vi "ProgramGS200andRun.vi"(5 "error in":errorcluster, 6 "Run program?":bool, 7 "Interval input":dbl, 8 "Slope Input":dbl, 9 "Voltage array":dbl[](array[numeric]), 10 "VISA resource name":refnum<visa-resource-name>) -> (0 "error out":errorcluster, 3 "VISA resource name out":refnum<visa-resource-name>)   [LabVIEW 2019]
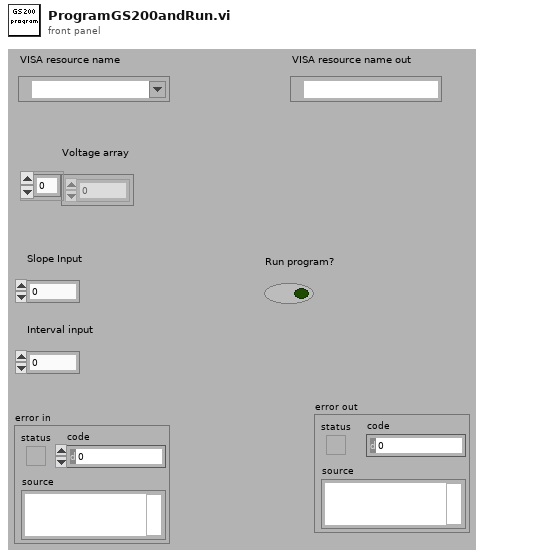
[diagram p1: front panel]
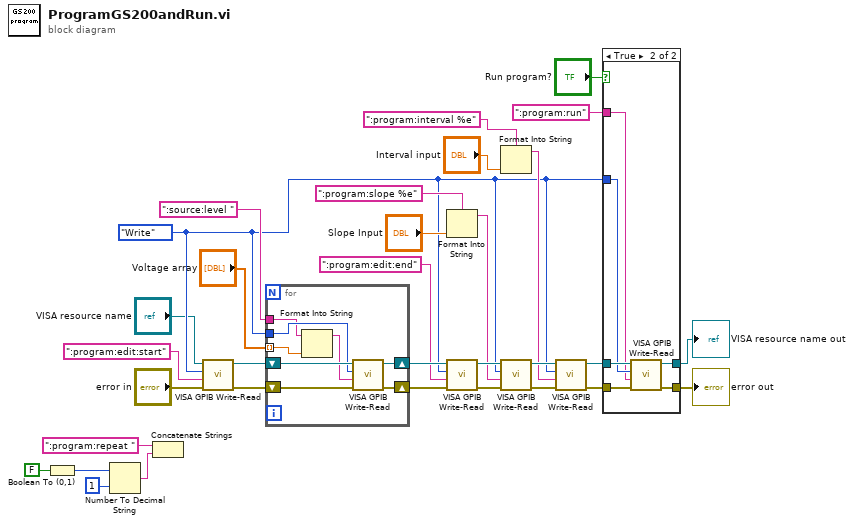
[diagram p0: block diagram]
diagram:
  w5 = enum16{"Write", "Read", "Write & Read"}."Write" ("Action")
  n1 = Boolean To (0,1)(Boolean=FALSE ("Repeat program?")) -> (0, 1=w25:i16)
  n2 = Number To Decimal String(number=w25, width (-)=i16 1) -> (decimal integer string=w22:string)
  n3 = Concatenate Strings(":program:repeat ", w22) -> ()  [unwired: 1 out]
  n4 = call "VISA GPIB Write-Read.vi"("error in (no error)"="error in", "Command"=":program:edit:start", "Action"=w5, "VISA resource name"="VISA resource name") -> ("error out"=w19:errorcluster, "dup VISA Session"=w20:refnum<visa-resource-name>)  [unwired: 4 in, 2 out]
  n5 = for {
    tunnel: ":source:level " -> [w36]
    tunnel: w5 -> [w38]
    tunnel: "Voltage array" -> [w35] mode=indexing
    shift-right: [w34] -> w15
    shift-left: w19 -> [w39]
    shift-right: [w33] -> w16
    shift-left: w20 -> [w40]
    n6 = Format Into String(initial string=w36, w35) -> (resulting string=w37:string)  [unwired: 2 in, 1 out]
    n7 = call "VISA GPIB Write-Read.vi"("error in (no error)"=w39, "Command"=w37, "Action"=w38, "VISA resource name"=w40) -> ("error out"=w34:errorcluster, "dup VISA Session"=w33:refnum<visa-resource-name>)  [unwired: 4 in, 2 out]
  }
  n8 = Format Into String(format string=":program:slope %e", "Slope Input") -> (resulting string=w11:string)  [unwired: 2 in, 1 out]
  n9 = call "VISA GPIB Write-Read.vi"("error in (no error)"=w15, "Command"=":program:edit:end", "Action"=w5, "VISA resource name"=w16) -> ("error out"=w12:errorcluster, "dup VISA Session"=w13:refnum<visa-resource-name>)  [unwired: 4 in, 2 out]
  n10 = Format Into String(format string=":program:interval %e", "Interval input") -> (resulting string=w8:string)  [unwired: 2 in, 1 out]
  n11 = call "VISA GPIB Write-Read.vi"("error in (no error)"=w12, "Command"=w11, "Action"=w5, "VISA resource name"=w13) -> ("error out"=w9:errorcluster, "dup VISA Session"=w10:refnum<visa-resource-name>)  [unwired: 4 in, 2 out]
  n12 = call "VISA GPIB Write-Read.vi"("error in (no error)"=w9, "Command"=w8, "Action"=w5, "VISA resource name"=w10) -> ("error out"=w6:errorcluster, "dup VISA Session"=w7:refnum<visa-resource-name>)  [unwired: 4 in, 2 out]
  n13 = case shown="True" "Run program?" {
    tunnel: w7 -> [w41 w48]
    tunnel: w6 -> [w42 w47]
    tunnel: w5 -> [_ w46]
    tunnel: [w42 w45] -> w26
    tunnel: ":program:run" -> [_ w44]
    tunnel: [w41 w43] -> w1
    frame False {
    }
    frame True {
      n14 = call "VISA GPIB Write-Read.vi"("error in (no error)"=w47, "Command"=w44, "Action"=w46, "VISA resource name"=w48) -> ("error out"=w45:errorcluster, "dup VISA Session"=w43:refnum<visa-resource-name>)  [unwired: 4 in, 2 out]
    }
  }
  "error out" <- w26
  "VISA resource name out" <- w1
